vi "BooleanCurrencyDataTypeHandling.vi"() -> ()   [LabVIEW 2019]
uses:
  <vilib>/Utility/error.llb/DialogType.ctl
  <vilib>/addons/database/Connection.llb/DB Tools Open Connec (String).vi
  <vilib>/addons/database/NI_Database_API.lvlib
panel:
  in  "Marks":dbl
  in  "Subject Name":string
  in  "Pass or Fail in exam":bool
  in  "Enter your Salary Here":dbl
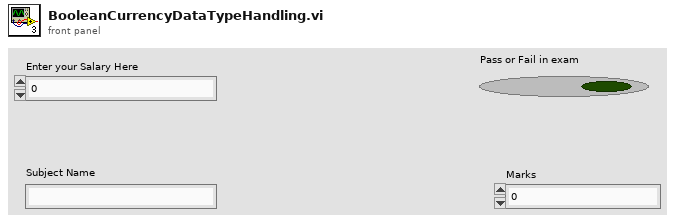
[diagram p1: front panel]
types:
  T1 = typedef "DialogType.ctl" = u16
  T2 = typedef "NI_Database_API.lvlib/Conn ObjectReference.ctl" = refnum<k1>
  T3 = cluster{string, string, "Subject Name ":string, "Marks":dbl}
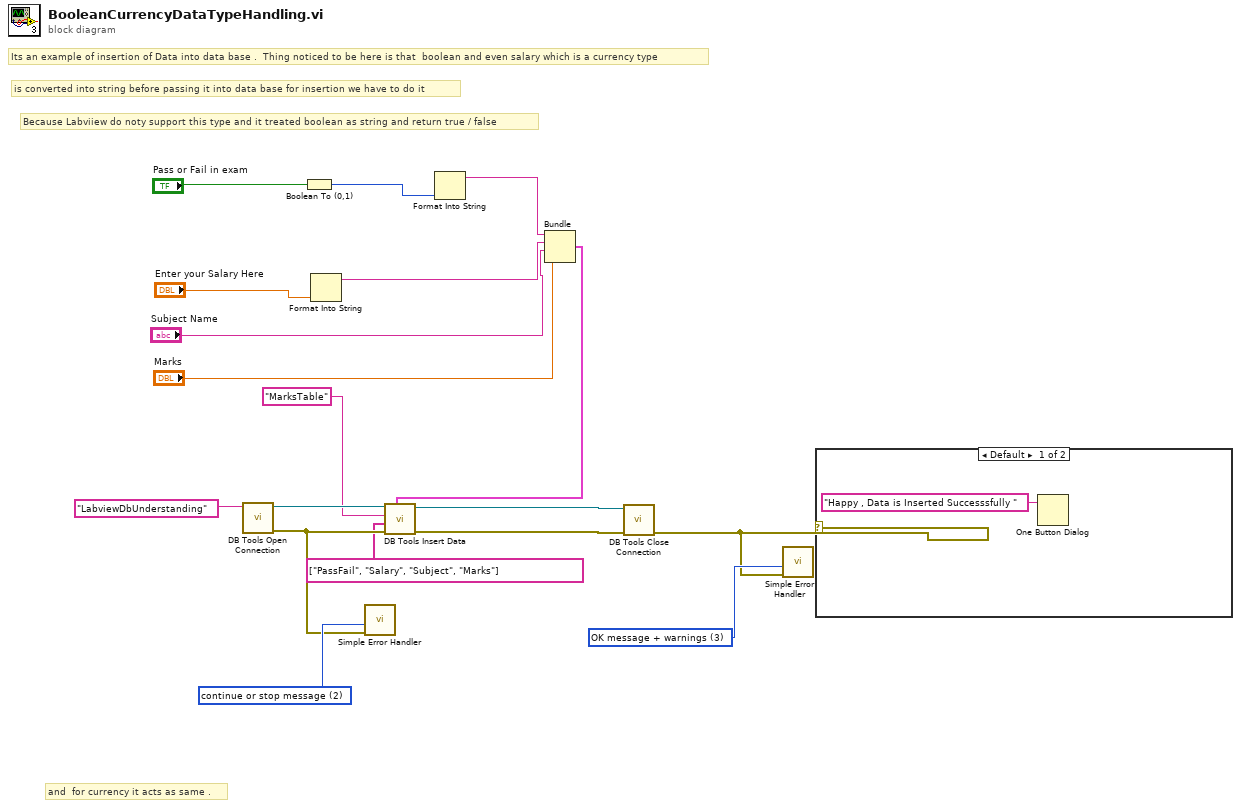
[diagram p0: block diagram]
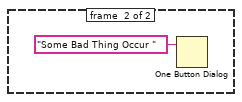
[diagram p2: hidden frame]
diagram:
  w11 = T1 3 items=["no dialog", "OK message", "continue or stop message", "OK message + warnings", "continue/stop + warnings"] ("type of dialog (OK msg:1)")
  w16 = T1 2 items=["no dialog", "OK message", "continue or stop message", "OK message + warnings", "continue/stop + warnings"] ("type of dialog (OK msg:1)")
  # "and  for currency it acts as same ."
  # "Because Labviiew do noty support this type and it treated boolean as string and return true / false"
  # "is converted into string before passing it into data base for insertion we have to do it"
  # "Its an example of insertion of Data into data base .  Thing noticed to be here is that  boolean and even salary which is a currency type"
  n1 = call-poly <vilib>:"DB Tools Open Connection.vi"("connection information"="LabviewDbUnderstanding") -> ("error out"=w15:errorcluster, "connection reference"=w17:T2)  [unwired: 7 in]
  n2 = Boolean To (0,1)(Boolean="Pass or Fail in exam") -> (0, 1=w8:i16)
  n3 = Format Into String("Enter your Salary Here") -> (resulting string=w5:string)  [unwired: 3 in, 1 out]
  n4 = call <vilib>:"Simple Error Handler.vi"("type of dialog (OK msg:1)"=w16, "error in (no error)"=w15) -> ()  [unwired: 3 in, 5 out]
  n5 = Format Into String(w8) -> (resulting string=w6:string)  [unwired: 3 in, 1 out]
  n6 = Bundle(w6, w5, "Subject Name"="Subject Name", "Marks"="Marks") -> (w4:T3)  [unwired: 1 in]
  n7 = call <vilib>:"DB Tools Insert Data.vi"("data"=w4, "error in (no error)"=w15, "columns"=string[] ["PassFail", "Salary", "Subject", "Marks"], "table"="MarksTable", "connection reference"=w17) -> ("error out"=w12:errorcluster, "connection reference out"=w13:T2)  [unwired: 5 in]
  n8 = call <vilib>:"DB Tools Close Connection.vi"("error in (no error)"=w12, "connection reference"=w13) -> ("error out"=w1:errorcluster)  [unwired: 5 in]
  n9 = call <vilib>:"Simple Error Handler.vi"("type of dialog (OK msg:1)"=w11, "error in (no error)"=w1) -> ()  [unwired: 3 in, 5 out]
  n10 = case shown="Default" w1 {
    frame #0 {
      n11 = One Button Dialog(message="Happy , Data is Inserted Successsfully ") -> ()  [unwired: 1 in, 1 out]
    }
    frame #1 {
      n12 = One Button Dialog(message="Some Bad Thing Occur ") -> ()  [unwired: 1 in, 1 out]
    }
  }
